vi "PDP Error= Message.vi"(0 "Message":string) -> ()   [LabVIEW 2010]
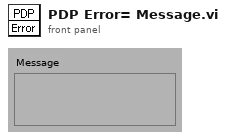
[diagram p1: front panel]
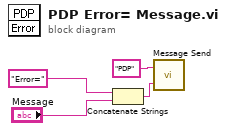
[diagram p0: block diagram]
diagram:
  n1 = Concatenate Strings("Error=", "Message") -> (w3:string)
  n2 = call "Message Send.vi"("Message"=w3, "Destination"="PDP") -> ()
